vi "PDP.vi"() -> ()   [LabVIEW 2010]
doc: "This VI represents about 90% of the user interface, the remainder consisting of the various pop-up windows.\nA diagram of the NMR system is presented, with buttons to represent each component. Parameters may be changed by pressing one of these buttons, which results in messages being passed to one of several other, high-level VIs whose job it is to take action. After such action is taken, messages may be passed back to this VI, indicating new data to be displayed on the front panel."
uses:
  PDP Global.vi
  TPS Global.vi
  <vilib>/Utility/config.llb/Read Key (Path).vi
  TMC-Target_Motion_Control/TMC Global.vi
  <vilib>/Utility/config.llb/NI_LVConfig.lvlib
panel:
  in  "Case Constant\n(See Context Help)":bool
  out "Collector Temp":dbl=9.54 format="%.1f"
  in  "RF Off":bool
  in  "RF On":bool
  in  "Mon. Time":i32=30
  in  "He4 Range":i32(ring)=2 items=["X 1", "X 0.1", "X 0.01", "X 0.001"]
  out "Polysub Signal":cluster{"x-Axis":dbl[], "Signal":dbl[]}(graph)
  out "CarbGlass":dbl=9.54
  out "Bottom Chip":dbl=9.54
  out "Top Chip":dbl=9.54
  out "NMR Tune Light":bool
  in  "NMR Tune":bool
  out "Clear Message Time":i32
  in  "DC Convert":bool
  out "Vacuum Pressure":dbl format="%.2e"
  out "Bot Plat (K)":dbl=nan format="%.1f"
  out "Top Plat (K)":dbl=nan format="%.1f"
  out "Motion Mask":bool
  in  "Submit Comment":bool
  out "DC Level (V)":dbl=9.54 format="%.3f"
  out "QMeter Temp":dbl=9.54 format="%.1f"
  in  "User Comment (press submit when done)":string
  out "HP Freq(GHz)":dbl=500.0 format="%.5f"
  out "Heater 2":bool
  in  "FM Offset (V)":dbl format="%.1f"
  in  "FM Amplitude (V)":dbl=3.0 format="%.1f"
  out "Power (mW)":dbl=500.0 format="%.3f"
  out "Freq (GHz)":dbl=500.0 format="%.3f"
  in  "Stop NMR Sweep":bool
  in  "Enable TCL Buttons":bool
  in  "NewEventFile":bool
  in  "NewBaseFile":bool
  out "LN2":dbl(slide) scale=0.0..100.0
  out "Magnet":dbl(slide) scale=0.0..100.0
  out "Separator Flow":dbl=10.0 format="%.1f"
  out "Main Flow":dbl=9.83 format="%.1f"
  in  "Beep on Update":bool
  out "Raw & Base":cluster{"x-Axis":dbl[], "Signal":dbl[]}[](graph)
  in  "Move Target":bool
  out "Encoder":dbl format="%.3f"
  out "Target Pos":i32(listbox)
  in  "5 min":bool
  out "History Plot":cluster{dbl, dbl}[](graph)
  out "Event Number":i32=-15
  in  "Scan Freq":i32=100
  in  "ScanSteps":i32=500
  in  "RF Power":i32=280
  in  "RF Mod":i32=400
  in  "Sweeps":i32=100
  in  "RF Freq":dbl=213.0 format="%.3f"
  in  "Yale Gain":i32(listbox)
  in  "Decrease":bool
  in  "Increase":bool
  in  "Up":bool
  in  "Down":bool
  in  "+1 hour":bool
  in  "30 min":bool
  in  "15 min":bool
  out "Polarization (%)":string="-13.06%"
  out "Monitor Light":bool
  in  "Monitor":bool
  out "Take Data Light":bool
  out "Pause Light":bool=TRUE
  out "QMeter":string="Bot Proton NH3"
  in  "Error":bool
  out "3He Pressure":dbl=9.83 format="%.3f"
  out "4He Pressure":dbl=-0.06 format="%.3f"
  in  "Magnet Lockout":bool
  in  "Heater Delay Done":dbl=2993221584.8599997 format="%.2f"
  out "Heater Delay":i8
  in  "To Zero":bool
  in  "Hold":bool
  in  "To Setpoint":bool
  in  "Switch Heater Off":bool
  out "Timestamp":string="06May1999  19h28m14s"
  in  "Init QCA":bool
  out "PolyFit Area (arb units)":dbl=-14.751 format="%.8f"
  out "User Message":string="Message: 23Jul2001  15h39m59s\nQCA Module Started"
  in  "Cal. Const.":dbl=0.64413 format="%.6f"
  in  "5T Superconducting Magnet":T1={"Current (A)"=77.15, "Witness (mT)"=77.15, "Field (T)"=77.15} {"Field (T)" format="%.2f"; "Witness (mT)" format="%.3f"; "Current (A)" format="%.3f"}
  out "Update At (sec)":i32=2147483647
  out "Next Update":i32=1151566443
  in  "Baseline":bool
  out "Heater 1":bool
  out "Magnet Power Supply":T2={"Current (A):"=0.0, "Voltage (V):"=-0.01, "Setpoint (A):"=77.15, "Rate (A/min):"=0.3, "Heater Status"="Persistent Mode", "Status:"=enum."Hold"} {"Rate (A/min):" format="%.3f"; "Setpoint (A):" format="%.3f"; "Voltage (V):" format="%.3f"; "Current (A):" format="%.3f"}
  out "Subtracted Signal & PolyFit Curve":cluster{"x-Axis":dbl[], "Signal":dbl[]}[](graph)
  out "3He Temp":dbl=1.023 format="%.2f"
  out "4He Temp":dbl=nan format="%.2f"
  in  "Save Channel List":bool
  in  "Switch Heater On":bool
  in  "Rate (A/min)":dbl=0.5 format="%.2f"
  in  "SetPoint (A)":dbl=77.085 format="%.3f"
  in  "NMR Channel":i32(listbox)
  in  "Previous Messages":u16(ring)
  in  "Take Data":bool
  in  "One Point":bool
  in  "Pause":bool
  # "Data for Last Event Displayed:"
  # "RF Output"
  # "X-Axis"
  # "-->"
  # "Y-Axis"
  # "<--"
  # "Temp (K)"
  # "Press (Torr)"
  # "Range"
  # "4He"
  # "3He"
  # "Top"
  # "Bottom"
  # "Chip (W)"
  # "Plat (K)"
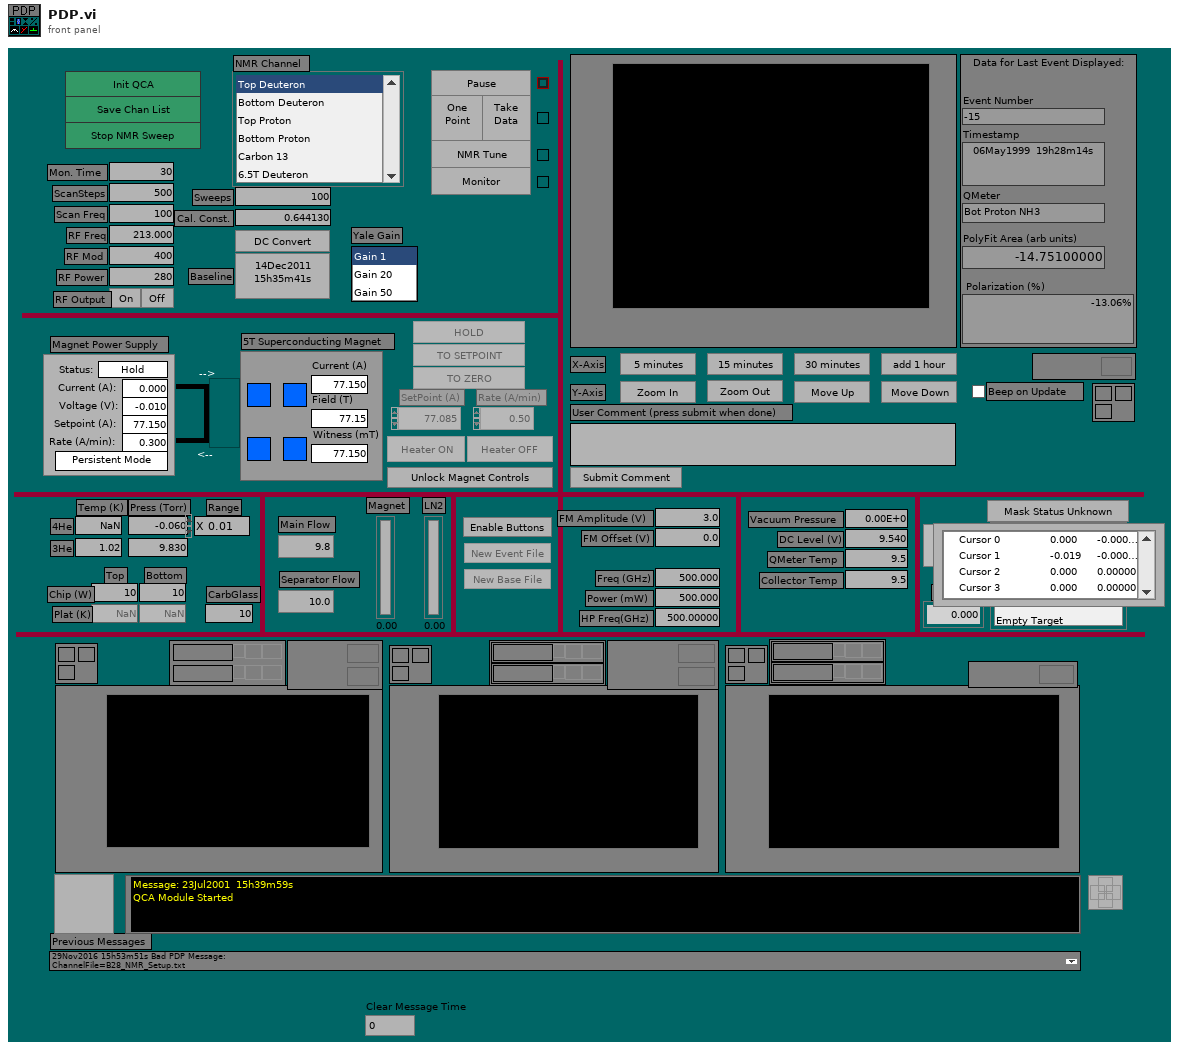
[diagram p1: front panel]
types:
  T1 = cluster{"Current (A)":dbl, "Witness (mT)":dbl, "Field (T)":dbl}
  T2 = cluster{"Current (A):":dbl, "Voltage (V):":dbl, "Setpoint (A):":dbl, "Rate (A/min):":dbl, "Heater Status":string, "Status:":enum16{"Hold", "To Setpoint", "To Zero", "Clamped"}}
  T3 = enum16{"No Message", "Bad Message", "RFFreq=", "RFMod=", "RFPower=", "QMeterName=", "YaleGain=", "ScanSweeps=", "ScanSteps=", "ScanFreq=", "Material=", "Baseline=", "CalConst=", "MonitorDelay=", "Channel=", "Channels=", "QCAPause", "QCATakeData", "QCANMRTune", "QCAMonitor", "Timer=", "LeadCurrent=", "LeadVoltage=", "MagCurrent=", "MagField=", "MagStatus=", "Setpoint=", "Setrate=", "HeaterDelay=", "Heater=", "HeaterDialog", "MagRemote", "MagLocal", "SendHe4Range", "uWaveFreq=", "uWavePower=", "BellowsPos=", "Event=", "Beep", "Message=", "Warning=", "Error=", "Address=", "Stop"}
  T4 = typedef "NI_LVConfig.lvlib/Config Data RefNum.ctl" = refnum<k1>
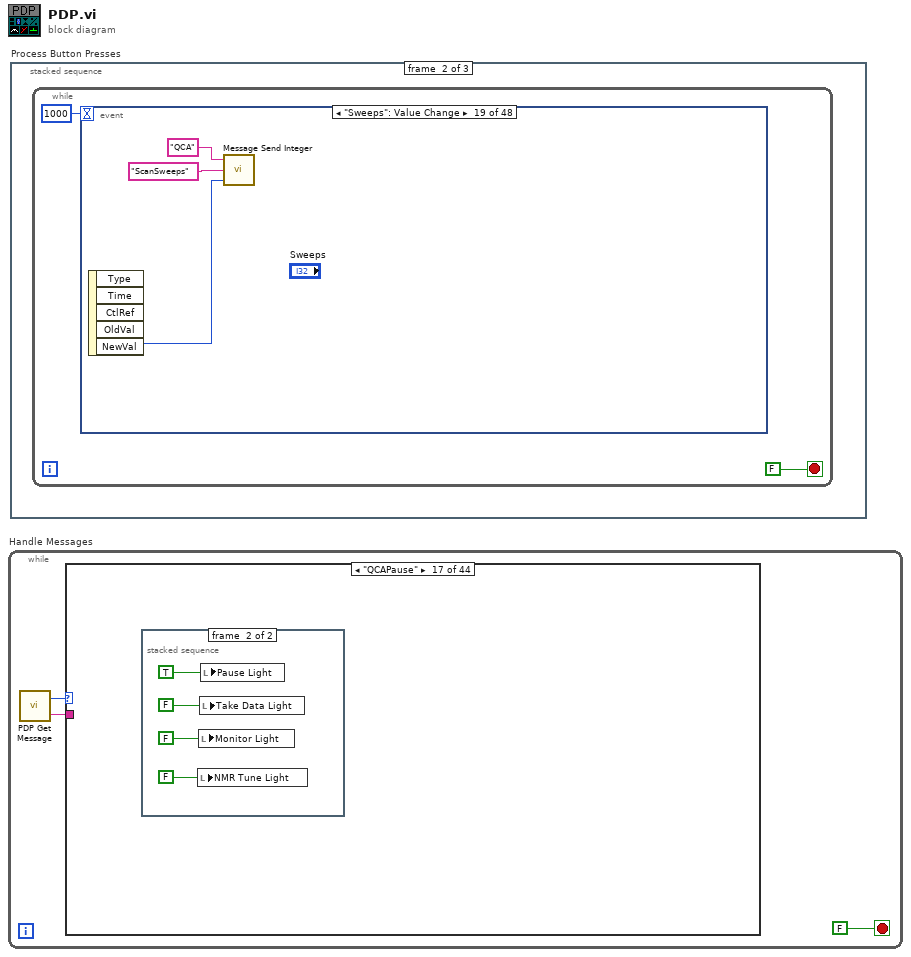
[diagram p0: block diagram]
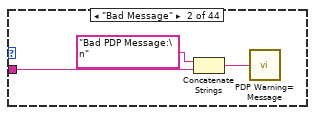
[diagram p3: hidden frame]
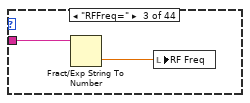
[diagram p4: hidden frame]
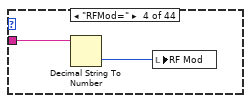
[diagram p5: hidden frame]
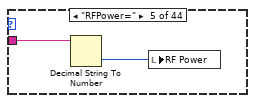
[diagram p6: hidden frame]
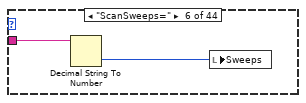
[diagram p7: hidden frame]
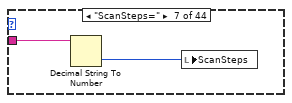
[diagram p8: hidden frame]
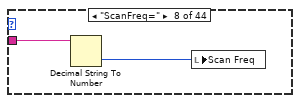
[diagram p9: hidden frame]
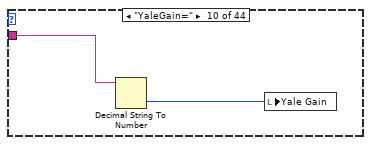
[diagram p11: hidden frame]
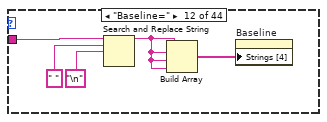
[diagram p13: hidden frame]
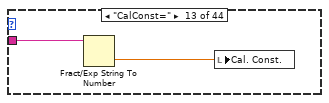
[diagram p14: hidden frame]
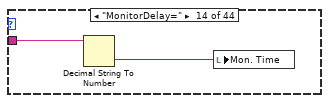
[diagram p15: hidden frame]
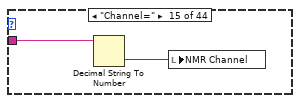
[diagram p16: hidden frame]
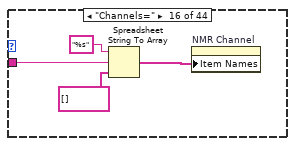
[diagram p17: hidden frame]
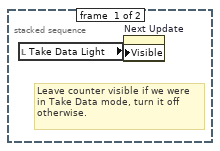
[diagram p18: hidden frame]
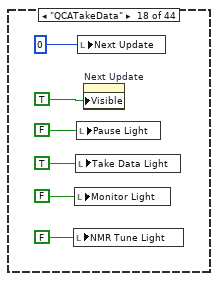
[diagram p19: hidden frame]
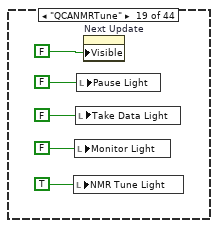
[diagram p20: hidden frame]
diagram:
  n1 = while "Handle Messages" {
    stop <- FALSE stop-if-true
    n2 = call "PDP Get Message.vi"() -> ("PDP Message Type"=w2:T3, "Text"=w3:string)  [unwired: 1 in]
    n3 = case shown="\"QCAPause\"" w2 {
      tunnel: w3 -> [_ w4 w8 w10 w12 w14 w16 w18 _ w20 _ w24 w27 w29 w31 w32 _ _ _ _ w61 w62 w66 w70 w74 w79 w83 w87 w94 w102 _ _ _ _ w126 w128 w130 w131 _ w396 w410 w425 w438 _]
      frame "No Message" {
      }
      frame "Bad Message" {
        n4 = Concatenate Strings("Bad PDP Message:\n" ("Message"), w4) -> (w5:string)
        n5 = call "PDP Warning= Message.vi"("Message"=w5) -> ()
      }
      frame "RFFreq=" {
        n6 = Fract/Exp String To Number(string=w8) -> (number=w7:dbl)  [unwired: 3 in, 1 out]
        n7 = local write "RF Freq"(w7) -> ()
      }
      frame "RFMod=" {
        n8 = Decimal String To Number(string=w10) -> (number=w9:i32)  [unwired: 2 in, 1 out]
        n9 = local write "RF Mod"(w9) -> ()
      }
      frame "RFPower=" {
        n10 = Decimal String To Number(string=w12) -> (number=w11:i32)  [unwired: 2 in, 1 out]
        n11 = local write "RF Power"(w11) -> ()
      }
      frame "ScanSweeps=" {
        n12 = Decimal String To Number(string=w14) -> (number=w13:i32)  [unwired: 2 in, 1 out]
        n13 = local write "Sweeps"(w13) -> ()
      }
      frame "ScanSteps=" {
        n14 = Decimal String To Number(string=w16) -> (number=w15:i32)  [unwired: 2 in, 1 out]
        n15 = local write "ScanSteps"(w15) -> ()
      }
      frame "ScanFreq=" {
        n16 = Decimal String To Number(string=w18) -> (number=w17:i32)  [unwired: 2 in, 1 out]
        n17 = local write "Scan Freq"(w17) -> ()
      }
      frame "QMeterName=" {
      }
      frame "YaleGain=" {
        n18 = Decimal String To Number(string=w20) -> (number=w19:i32)  [unwired: 2 in, 1 out]
        n19 = local write "Yale Gain"(w19) -> ()
      }
      frame "Material=" {
      }
      frame "Baseline=" {
        n20 = Search and Replace String(input string=w24, search string=" ", replace string="\n" ("replace string (\"\")")) -> (result string=w21:string)  [unwired: 5 in, 3 out]
        n21 = Build Array(w21, w21, w21, w21) -> (w25:string[])
        n22 = property on="Baseline" class="Bool"("Strings [4]"=w25) -> ()  [unwired: 2 in, 2 out]
      }
      frame "CalConst=" {
        n23 = Fract/Exp String To Number(string=w27) -> (number=w26:dbl)  [unwired: 3 in, 1 out]
        n24 = local write "Cal. Const."(w26) -> ()
      }
      frame "MonitorDelay=" {
        n25 = Decimal String To Number(string=w29) -> (number=w28:i32)  [unwired: 2 in, 1 out]
        n26 = local write "Mon. Time"(w28) -> ()
      }
      frame "Channel=" {
        n27 = Decimal String To Number(string=w31) -> (number=w30:i32)  [unwired: 2 in, 1 out]
        n28 = local write "NMR Channel"(w30) -> ()
      }
      frame "Channels=" {
        n29 = Spreadsheet String To Array(format string="%s", spreadsheet string=w32, array type (2D Dbl)=string[] []) -> (array=w34:string[])  [unwired: 1 in]
        n30 = property on="NMR Channel" class="LstBox (strict)"("Item Names"=w34) -> ()  [unwired: 2 in, 2 out]
      }
      frame "QCAPause" {
        n31 = stacked-sequence {
          frame #0 {
            # "Leave counter visible if we were\nin Take Data mode, turn it off\notherwise."
            n32 = local read "Take Data Light"() -> (w36:bool)
            n33 = property on="Next Update" class="DigNum (strict)"("Visible"=w36) -> ()  [unwired: 2 in, 2 out]
          }
          frame #1 {
            n34 = local write "NMR Tune Light"(FALSE ("NMR Tune Light")) -> ()
            n35 = local write "Monitor Light"(FALSE ("Cont Sweep Light")) -> ()
            n36 = local write "Take Data Light"(FALSE ("Take Data Light")) -> ()
            n37 = local write "Pause Light"(TRUE ("Pause Light")) -> ()
          }
        }
      }
      frame "QCATakeData" {
        n38 = local write "NMR Tune Light"(FALSE ("NMR Tune Light")) -> ()
        n39 = local write "Monitor Light"(FALSE ("Cont Sweep Light")) -> ()
        n40 = local write "Take Data Light"(TRUE ("Take Data Light")) -> ()
        n41 = local write "Pause Light"(FALSE ("Pause Light")) -> ()
        n42 = local write "Next Update"(0 ("Next Update")) -> ()
        n43 = property on="Next Update" class="DigNum (strict)"("Visible"=TRUE) -> ()  [unwired: 2 in, 2 out]
      }
      frame "QCANMRTune" {
        n44 = local write "NMR Tune Light"(TRUE ("NMR Tune Light")) -> ()
        n45 = local write "Monitor Light"(FALSE ("Cont Sweep Light")) -> ()
        n46 = local write "Take Data Light"(FALSE ("Take Data Light")) -> ()
        n47 = local write "Pause Light"(FALSE ("Pause Light")) -> ()
        n48 = property on="Next Update" class="DigNum (strict)"("Visible"=FALSE) -> ()  [unwired: 2 in, 2 out]
      }
      frame "QCAMonitor" {
        n49 = local write "NMR Tune Light"(FALSE ("NMR Tune Light")) -> ()
        n50 = local write "Monitor Light"(TRUE ("Cont Sweep Light")) -> ()
        n51 = local write "Take Data Light"(FALSE ("Take Data Light")) -> ()
        n52 = local write "Pause Light"(FALSE ("Pause Light")) -> ()
        n53 = local write "Next Update"(0 ("Next Update")) -> ()
        n54 = property on="Next Update" class="DigNum (strict)"("Visible"=TRUE) -> ()  [unwired: 2 in, 2 out]
      }
      frame "Timer=" {
        n55 = Decimal String To Number(string=w61) -> (number=w59:i32)  [unwired: 2 in, 1 out]
        n56 = call "Get UNIX Time.vi"() -> ("UNIX seconds"=w60:i32)
        n57 = Add(x=w59, y=w60) -> (x+y=→"Update At (sec)":i32)
      }
      frame "LeadCurrent=" {
        n58 = Fract/Exp String To Number(string=w62) -> (number=w65:dbl)  [unwired: 3 in, 1 out]
        n59 = local read "Magnet Power Supply"() -> (w63:T2)
        n60 = Bundle By Name(cluster=w63, "Current (A):"=w65) -> (w64:T2)
        n61 = local write "Magnet Power Supply"(w64) -> ()
      }
      frame "LeadVoltage=" {
        n62 = Fract/Exp String To Number(string=w66) -> (number=w69:dbl)  [unwired: 3 in, 1 out]
        n63 = local read "Magnet Power Supply"() -> (w67:T2)
        n64 = Bundle By Name(cluster=w67, "Voltage (V):"=w69) -> (w68:T2)
        n65 = local write "Magnet Power Supply"(w68) -> ()
      }
      frame "MagCurrent=" {
        n66 = Fract/Exp String To Number(string=w70) -> (number=w71:dbl)  [unwired: 3 in, 1 out]
        n67 = local read "5T Superconducting Magnet"() -> (w73:T1)
        n68 = Bundle By Name(cluster=w73, "Current (A)"=w71) -> (w72:T1)
        n69 = local write "5T Superconducting Magnet"(w72) -> ()
      }
      frame "MagField=" {
        n70 = Fract/Exp String To Number(string=w74) -> (number=w75:dbl)  [unwired: 3 in, 1 out]
        n71 = local read "5T Superconducting Magnet"() -> (w77:T1)
        n72 = Bundle By Name(cluster=w77, "Field (T)"=w75) -> (w76:T1)
        n73 = local write "5T Superconducting Magnet"(w76) -> ()
      }
      frame "MagStatus=" {
        n74 = Decimal String To Number(string=w79) -> (number=w78:i32)  [unwired: 2 in, 1 out]
        n75 = local read "Magnet Power Supply"() -> (w80:T2)
        n76 = Bundle By Name(cluster=w80, "Status:"=w78) -> (→"Magnet Power Supply":T2)
      }
      frame "Setpoint=" {
        n77 = Fract/Exp String To Number(string=w83) -> (number=w82:dbl)  [unwired: 3 in, 1 out]
        n78 = local write "SetPoint (A)"(w82) -> ()
        n79 = global write "PDP Global.vi" "Setpoint"(w82) -> ()
        n80 = local read "Magnet Power Supply"() -> (w84:T2)
        n81 = Bundle By Name(cluster=w84, "Setpoint (A):"=w82) -> (w85:T2)
        n82 = local write "Magnet Power Supply"(w85) -> ()
      }
      frame "Setrate=" {
        n83 = Fract/Exp String To Number(string=w87) -> (number=w86:dbl)  [unwired: 3 in, 1 out]
        n84 = local write "Rate (A/min)"(w86) -> ()
        n85 = global write "PDP Global.vi" "Setrate"(w86) -> ()
        n86 = local read "Magnet Power Supply"() -> (w88:T2)
        n87 = Bundle By Name(cluster=w88, "Rate (A/min):"=w86) -> (w89:T2)
        n88 = local write "Magnet Power Supply"(w89) -> ()
      }
      frame "HeaterDelay=" {
        n89 = Decimal String To Number(string=w94) -> (number=w91:i32)  [unwired: 2 in, 1 out]
        n90 = Get Date/Time In Seconds() -> (seconds since 1Jan1904=w90:timestamp)
        n91 = To Double Precision Float(number=w90) -> (double precision float=w93:dbl)
        n92 = Add(x=w91, y=w93) -> (x+y=w92:dbl)
        n93 = stacked-sequence {
          tunnel: w92 -> [w96 _]
          tunnel: w91 -> [w95 _]
          frame #0 {
            n94 = local write "Heater Delay Done"(w96) -> ()
            n95 = local write "Heater Delay"(w95) -> ()
          }
          frame #1 {
            n96 = property on="Switch Heater On" class="Bool"("Visible"=FALSE) -> ()  [unwired: 2 in, 2 out]
            n97 = property on="Switch Heater Off" class="Bool"("Visible"=FALSE) -> ()  [unwired: 2 in, 2 out]
            n98 = property on="Heater Delay" class="DigNum (strict)"("Visible"=TRUE) -> ()  [unwired: 2 in, 2 out]
          }
        }
      }
      frame "Heater=" {
        n99 = To Upper Case(1:w102) -> (0:w100:string)
        n100 = Equal?(x="ON", y=w100) -> (x = y?=w101:bool)
        "Heater 1" <- w101
        "Heater 2" <- w101
        n101 = Select(t="Driven Mode", s=w101, f="Persistent Mode") -> (s? t:f=w108:string)
        n102 = local read "Magnet Power Supply"() -> (w103:T2)
        n103 = Bundle By Name(cluster=w103, "Heater Status"=w108) -> (w104:T2)
        n104 = local write "Magnet Power Supply"(w104) -> ()
      }
      frame "HeaterDialog" {
        n105 = Two Button Dialog(message="Are you sure you want to turn the switch heater on? ", 1:"Cancel - No Change" ("F button name (\"Cancel\")"), 2:"Turn Heater On" ("T button name (\"OK\")")) -> (T button?=w109:bool)
        n106 = case shown="True" w109 {
          frame False {
          }
          frame True {
            n107 = call "Message Send Text.vi"("Value"="On,Confirm" ("Message"), "Parameter"="Heater", "Destination"="SMC") -> ()
          }
        }
      }
      frame "MagRemote" {
        w116 = u8 0
        n108 = Build Array("Lock Magnet Controls") -> (w118:string[])
        n109 = property on="SetPoint (A)" class="DigNum (strict)"("Disabled"=w116) -> ()  [unwired: 2 in, 2 out]
        n110 = property on="Switch Heater On" class="Bool"("Disabled"=w116) -> ()  [unwired: 2 in, 2 out]
        n111 = property on="Switch Heater Off" class="Bool"("Disabled"=w116) -> ()  [unwired: 2 in, 2 out]
        n112 = property on="Magnet Lockout" class="Bool"("Strings [4]"=w118) -> ()  [unwired: 2 in, 2 out]
        n113 = property on="Rate (A/min)" class="DigNum (strict)"("Disabled"=w116) -> ()  [unwired: 2 in, 2 out]
        n114 = property on="Hold" class="Bool"("Disabled"=w116) -> ()  [unwired: 2 in, 2 out]
        n115 = property on="To Setpoint" class="Bool"("Disabled"=w116) -> ()  [unwired: 2 in, 2 out]
        n116 = property on="To Zero" class="Bool"("Disabled"=w116) -> ()  [unwired: 2 in, 2 out]
      }
      frame "MagLocal" {
        w119 = u8 2
        n117 = Build Array("Unlock Magnet Controls") -> (w121:string[])
        n118 = property on="SetPoint (A)" class="DigNum (strict)"("Disabled"=w119) -> ()  [unwired: 2 in, 2 out]
        n119 = property on="Switch Heater On" class="Bool"("Disabled"=w119) -> ()  [unwired: 2 in, 2 out]
        n120 = property on="Switch Heater Off" class="Bool"("Disabled"=w119) -> ()  [unwired: 2 in, 2 out]
        n121 = property on="Magnet Lockout" class="Bool"("Strings [4]"=w121) -> ()  [unwired: 2 in, 2 out]
        n122 = property on="Rate (A/min)" class="DigNum (strict)"("Disabled"=w119) -> ()  [unwired: 2 in, 2 out]
        n123 = property on="Hold" class="Bool"("Disabled"=w119) -> ()  [unwired: 2 in, 2 out]
        n124 = property on="To Setpoint" class="Bool"("Disabled"=w119) -> ()  [unwired: 2 in, 2 out]
        n125 = property on="To Zero" class="Bool"("Disabled"=w119) -> ()  [unwired: 2 in, 2 out]
      }
      frame "SendHe4Range" {
        n126 = call "Message Send Integer.vi"("Value"="He4 Range", "Parameter"="He4Range", "Destination"="TTM") -> ()
      }
      frame "uWaveFreq=" {
        n127 = Fract/Exp String To Number(string=w126) -> (number=w125:dbl)  [unwired: 3 in, 1 out]
        n128 = local write "Freq (GHz)"(w125) -> ()
      }
      frame "uWavePower=" {
        n129 = Fract/Exp String To Number(string=w128) -> (number=w127:dbl)  [unwired: 3 in, 1 out]
        n130 = local write "Power (mW)"(w127) -> ()
      }
      frame "BellowsPos=" {
        n131 = Fract/Exp String To Number(string=w130) -> (number=w129:dbl)  [unwired: 3 in, 1 out]
        n132 = local write "HP Freq(GHz)"(w129) -> ()
      }
      frame "Event=" {
        n133 = Unflatten From String(type=string[][] [], binary string=w131) -> (value=w133:string[][])  [unwired: 3 in, 2 out]
        n134 = stacked-sequence {
          tunnel: w133 -> [w144 w172 w193 w200 w203 w207 w234 w237 w242 w246 w250 w255 w266 w275 w278 w282 w286 w290 w296 w302 w306 w310 w316 w322 w326 w335 w344 w348 w352 w359 w374 _ w391]
          frame #0 {
            # "Set the X axis of the signal plots."
            n135 = call "Text Get Event Fragment.vi"("Event"=w144, "Fragment Type"="RFFreq") -> ("Fragment"=w149:string)  [unwired: 1 out]
            n136 = call "Text Get Event Fragment.vi"("Event"=w144, "Fragment Type"="RFMod") -> ("Fragment"=w150:string)  [unwired: 1 out]
            n137 = call "Text Get Event Fragment.vi"("Event"=w144, "Fragment Type"="ScanSteps") -> ("Fragment"=w146:string)  [unwired: 1 out]
            n138 = global read "PDP Global.vi" "Last Mod"() -> (w140:dbl)
            n139 = global read "PDP Global.vi" "Last Freq"() -> (w143:dbl)
            n140 = global read "PDP Global.vi" "Last Steps"() -> (w141:i32)
            n141 = Fract/Exp String To Number(string=w149) -> (number=w142:dbl)  [unwired: 3 in, 1 out]
            n142 = Decimal String To Number(string=w150) -> (number=w148:i32)  [unwired: 2 in, 1 out]
            n143 = Decimal String To Number(string=w146) -> (number=w138:i32)  [unwired: 2 in, 1 out]
            n144 = Divide(x=w148, y=1000) -> (x/y=w139:dbl)
            n145 = Not Equal?(x=w143, y=w142) -> (x != y?=w135:bool)
            n146 = Not Equal?(x=w140, y=w139) -> (x != y?=w136:bool)
            n147 = Not Equal?(x=w141, y=w138) -> (x != y?=w137:bool)
            n148 = Compound Arithmetic op=OR(w135, w136, w137) -> (w134:bool)
            n149 = case shown="True" w134 {
              tunnel: w138 -> [_ w155]
              tunnel: w139 -> [_ w154]
              tunnel: w142 -> [_ w153]
              frame False {
              }
              frame True {
                n150 = global write "PDP Global.vi" "Last Mod"(w154) -> ()
                n151 = global write "PDP Global.vi" "Last Freq"(w153) -> ()
                n152 = global write "PDP Global.vi" "Last Steps"(w155) -> ()
                n153 = for {
                  N: w155 -> [_]
                  tunnel: [w163] -> w158 mode=indexing
                  i -> [w163]
                }
                n154 = Multiply(x=w158, y=2) -> (x*y=w159:i32[])
                n155 = Divide(x=w159, y=w155) -> (x/y=w162:dbl[])
                n156 = Decrement(x=w162) -> (x-1=w156:dbl[])
                n157 = Multiply(x=w154, y=w156) -> (x*y=w161:dbl[])
                n158 = Add(x=w153, y=w161) -> (x+y=w160:dbl[])
                n159 = global write "PDP Global.vi" "x-Axis"(w160) -> ()
              }
            }
          }
          frame #1 {
            # "Display the Raw Signal and the Baseline Signal."
            n160 = call "Text Get Event Fragment.vi"("Event"=w172, "Fragment Type"="RawSignal") -> ("Fragment"=w171:string)  [unwired: 1 out]
            n161 = call "Text Get Event Fragment.vi"("Event"=w172, "Fragment Type"="BaseSignal") -> ("Fragment"=w170:string)  [unwired: 1 out]
            n162 = global read "PDP Global.vi" "x-Axis"() -> (w168:dbl[])
            n163 = call "String 2 Signal.vi"("String"=w171) -> ("Signal"=w165:dbl[])
            n164 = call "String 2 Signal.vi"("String"=w170) -> ("Signal"=w167:dbl[])
            n165 = Array Size(array=w167) -> (size(s)=w169:i32)
            n166 = Greater Than 0?(x=w169) -> (x > 0?=w164:bool)
            n167 = case shown="True" w164 {
              tunnel: w168 -> [w178 w179]
              tunnel: w167 -> [_ w184]
              tunnel: [w175 w181] -> w166
              tunnel: w165 -> [w177 w180]
              frame False {
                n168 = Bundle("x-Axis"=w178, "Signal"=w177) -> (w176:cluster{"x-Axis":dbl[], "Signal":dbl[]})  [unwired: 1 in]
                n169 = Build Array(w176) -> (w175:cluster{"x-Axis":dbl[], "Signal":dbl[]}[])
              }
              frame True {
                n170 = Bundle("x-Axis"=w179, "Signal"=w180) -> (w183:cluster{"x-Axis":dbl[], "Signal":dbl[]})  [unwired: 1 in]
                n171 = Bundle("x-Axis"=w179, "Signal"=w184) -> (w182:cluster{"x-Axis":dbl[], "Signal":dbl[]})  [unwired: 1 in]
                n172 = Build Array(w183, w182) -> (w181:cluster{"x-Axis":dbl[], "Signal":dbl[]}[])
              }
            }
            "Raw & Base" <- w166
          }
          frame #2 {
            # "Display the Subtracted Signal and the Polyfit Curve."
            n173 = call "Text Get Event Fragment.vi"("Event"=w193, "Fragment Type"="SubSignal") -> ("Fragment"=w191:string)  [unwired: 1 out]
            n174 = call "Text Get Event Fragment.vi"("Event"=w193, "Fragment Type"="PolyCurve") -> ("Fragment"=w192:string)  [unwired: 1 out]
            n175 = global read "PDP Global.vi" "x-Axis"() -> (w188:dbl[])
            n176 = call "String 2 Signal.vi"("String"=w191) -> ("Signal"=w185:dbl[])
            n177 = call "String 2 Signal.vi"("String"=w192) -> ("Signal"=w189:dbl[])
            n178 = Bundle("x-Axis"=w188, "Signal"=w185) -> (w186:cluster{"x-Axis":dbl[], "Signal":dbl[]})  [unwired: 1 in]
            n179 = Bundle("x-Axis"=w188, "Signal"=w189) -> (w187:cluster{"x-Axis":dbl[], "Signal":dbl[]})  [unwired: 1 in]
            n180 = Build Array(w186, w187) -> (→"Subtracted Signal & PolyFit Curve":cluster{"x-Axis":dbl[], "Signal":dbl[]}[])
          }
          frame #3 {
            # "Display the Polysubtracted Signal."
            n181 = call "Text Get Event Fragment.vi"("Event"=w200, "Fragment Type"="PolySignal") -> ("Fragment"=w196:string)  [unwired: 1 out]
            n182 = global read "PDP Global.vi" "x-Axis"() -> (w199:dbl[])
            n183 = call "String 2 Signal.vi"("String"=w196) -> ("Signal"=w197:dbl[])
            n184 = Bundle("x-Axis"=w199, "Signal"=w197) -> (→"Polysub Signal":cluster{"x-Axis":dbl[], "Signal":dbl[]})  [unwired: 1 in]
          }
          frame #4 {
            # "Display the Polysubtracted Signal."
            n185 = call "Text Get Event Fragment.vi"("Event"=w203, "Fragment Type"="Area") -> ("Fragment"=w204:string)  [unwired: 1 out]
            n186 = Fract/Exp String To Number(string=w204) -> (number=→"PolyFit Area (arb units)":dbl)  [unwired: 3 in, 1 out]
          }
          frame #5 {
            # "Display the Polysubtracted Signal."
            n187 = call "Text Get Event Fragment.vi"("Event"=w207, "Fragment Type"="Polarization") -> ("Fragment"=w213:string, "Found"=w206:bool)
            n188 = call "Text Get Event Fragment.vi"("Event"=w207, "Fragment Type"="EventNum") -> ("Fragment"=w209:string)  [unwired: 1 out]
            n189 = Decimal String To Number(string=w209) -> (number=w208:i32)  [unwired: 2 in, 1 out]
            n190 = Fract/Exp String To Number(string=w213) -> (number=w211:dbl)  [unwired: 3 in, 1 out]
            n191 = case shown="True" w206 {
              tunnel: w211 -> [_ w218]
              tunnel: w208 -> [_ w219]
              frame False {
                n192 = local write "Polarization (%)"("") -> ()
              }
              frame True {
                n193 = call "UNIX to LabVIEW.vi"("UNIX Time"=w219) -> ("LabVIEW Time"=w220:dbl)
                n194 = Absolute Value(x=w218) -> (abs(x)=w217:dbl)
                n195 = property on="History Plot" class="XYGraph (strict)"() -> ("X Scale.Range:Maximum"=w223:dbl, "X Scale.Range:Minimum"=w226:dbl)  [unwired: 2 in, 2 out]
                n196 = Less?(x=w217, y=101.0) -> (x < y?=w215:bool)
                n197 = Format Into String(format string="%+6.1f%", w218) -> (resulting string=→"Polarization (%)":string)  [unwired: 2 in, 1 out]
                n198 = case shown="True" w215 {
                  tunnel: w220 -> [_ w229]
                  tunnel: w218 -> [_ w228]
                  frame False {
                    # "Glitch Signal - don't plot in strip chart"
                  }
                  frame True {
                    n199 = local read "History Plot"() -> (w232:cluster{dbl, dbl}[])
                    n200 = Bundle("LabVIEW Time"=w229, w228) -> (w230:cluster{"LabVIEW Time":dbl, dbl})  [unwired: 1 in]
                    n201 = Build Array (concatenate)(w230, w232) -> (→"History Plot":cluster{"LabVIEW Time":dbl, dbl}[])
                  }
                }
                n202 = Subtract(x=w220, y=w223) -> (x-y=w227:dbl)
                n203 = Compound Arithmetic op=ADD(w227, w223) -> (w225:dbl)
                n204 = Compound Arithmetic op=ADD(w227, w226) -> (w224:dbl)
                n205 = property on="History Plot" class="XYGraph (strict)"("X Scale.Range:Maximum"=w225, "X Scale.Range:Minimum"=w224) -> ()  [unwired: 2 in, 2 out]
              }
            }
          }
          frame #6 {
            # "Display the Polysubtracted Signal."
            n206 = call "Text Get Event Fragment.vi"("Event"=w234, "Fragment Type"="QMeterName") -> ("Fragment"=→"QMeter":string)  [unwired: 1 out]
          }
          frame #7 {
            n207 = call "Text Get Event Fragment.vi"("Event"=w237, "Fragment Type"="EventNum") -> ("Fragment"=w238:string)  [unwired: 1 out]
            n208 = Decimal String To Number(string=w238) -> (number=w236:i32)  [unwired: 2 in, 1 out]
            "Event Number" <- w236
            n209 = call "UNIX to Timestamp.vi"("Seconds"=w236) -> ("Timestamp String"=→"Timestamp":string)
          }
          frame #8 {
            # "Display the Polysubtracted Signal."
            n210 = call "Text Get Event Fragment.vi"("Event"=w242, "Fragment Type"="He3Press") -> ("Fragment"=w243:string)  [unwired: 1 out]
            n211 = Fract/Exp String To Number(string=w243) -> (number=→"3He Pressure":dbl)  [unwired: 3 in, 1 out]
          }
          frame #9 {
            # "Display the Polysubtracted Signal."
            n212 = call "Text Get Event Fragment.vi"("Event"=w246, "Fragment Type"="He3Temp") -> ("Fragment"=w247:string)  [unwired: 1 out]
            n213 = Fract/Exp String To Number(string=w247) -> (number=→"3He Temp":dbl)  [unwired: 3 in, 1 out]
          }
          frame #10 {
            # "Display the Polysubtracted Signal."
            n214 = call "Text Get Event Fragment.vi"("Event"=w250, "Fragment Type"="He4Press") -> ("Fragment"=w251:string)  [unwired: 1 out]
            n215 = Fract/Exp String To Number(string=w251) -> (number=→"4He Pressure":dbl)  [unwired: 3 in, 1 out]
          }
          frame #11 {
            # "Display the Polysubtracted Signal."
            n216 = call "Text Get Event Fragment.vi"("Event"=w255, "Fragment Type"="He4Temp") -> ("Fragment"=w256:string, "Found"=w253:bool)
            n217 = Fract/Exp String To Number(string=w256) -> (number=w254:dbl)  [unwired: 3 in, 1 out]
            n218 = case shown="True" w253 {
              tunnel: w254 -> [_ w258]
              frame False {
              }
              frame True {
                "4He Temp" <- w258
              }
            }
          }
          frame #12 {
            # "Display the Polysubtracted Signal."
            n219 = call "Text Get Event Fragment.vi"("Event"=w266, "Fragment Type"="TopPlat") -> ("Fragment"=w261:string)  [unwired: 1 out]
            n220 = Fract/Exp String To Number(string=w261) -> (number=w260:dbl)  [unwired: 3 in, 1 out]
            "Top Plat (K)" <- w260
            n221 = Less?(x=w260, y=49.0) -> (x < y?=w265:bool)
            n222 = Select(t=2, s=w265, f=0) -> (s? t:f=w262:i32)
            n223 = property on="Top Plat (K)" class="DigNum (strict)"("Disabled"=w262) -> ()  [unwired: 2 in, 2 out]
          }
          frame #13 {
            # "Display the Polysubtracted Signal."
            n224 = call "Text Get Event Fragment.vi"("Event"=w275, "Fragment Type"="BotPlat") -> ("Fragment"=w271:string)  [unwired: 1 out]
            n225 = Fract/Exp String To Number(string=w271) -> (number=w268:dbl)  [unwired: 3 in, 1 out]
            "Bot Plat (K)" <- w268
            n226 = Less?(x=w268, y=49.0) -> (x < y?=w274:bool)
            n227 = Select(t=2, s=w274, f=0) -> (s? t:f=w269:i32)
            n228 = property on="Bot Plat (K)" class="DigNum (strict)"("Disabled"=w269) -> ()  [unwired: 2 in, 2 out]
          }
          frame #14 {
            # "Display the Polysubtracted Signal."
            n229 = call "Text Get Event Fragment.vi"("Event"=w278, "Fragment Type"="uWaveFreq") -> ("Fragment"=w279:string)  [unwired: 1 out]
            n230 = Fract/Exp String To Number(string=w279) -> (number=→"Freq (GHz)":dbl)  [unwired: 3 in, 1 out]
          }
          frame #15 {
            # "Display the Polysubtracted Signal."
            n231 = call "Text Get Event Fragment.vi"("Event"=w282, "Fragment Type"="uWavePower") -> ("Fragment"=w283:string)  [unwired: 1 out]
            n232 = Fract/Exp String To Number(string=w283) -> (number=→"Power (mW)":dbl)  [unwired: 3 in, 1 out]
          }
          frame #16 {
            # "Display the Polysubtracted Signal."
            n233 = call "Text Get Event Fragment.vi"("Event"=w286, "Fragment Type"="HPFreq") -> ("Fragment"=w287:string)  [unwired: 1 out]
            n234 = Fract/Exp String To Number(string=w287) -> (number=→"HP Freq(GHz)":dbl)  [unwired: 3 in, 1 out]
          }
          frame #17 {
            n235 = call "Text Get Event Fragment.vi"("Event"=w290, "Fragment Type"="MainFlow") -> ("Fragment"=w291:string)  [unwired: 1 out]
            n236 = Fract/Exp String To Number(string=w291) -> (number=→"Main Flow":dbl)  [unwired: 3 in, 1 out]
          }
          frame #18 {
            n237 = call "Text Get Event Fragment.vi"("Event"=w296, "Fragment Type"="SepFlow") -> ("Fragment"=w297:string)  [unwired: 1 out]
            n238 = Fract/Exp String To Number(string=w297) -> (number=w294:dbl)  [unwired: 3 in, 1 out]
            "Separator Flow" <- w294
            n239 = Less?(x=w294, y=7.0) -> (x < y?=w295:bool)
            n240 = property on="Separator Flow" class="DigNum (strict)"("Blinking"=w295) -> ()  [unwired: 2 in, 2 out]
          }
          frame #19 {
            n241 = call "Text Get Event Fragment.vi"("Event"=w302, "Fragment Type"="Collector") -> ("Fragment"=w303:string)  [unwired: 1 out]
            n242 = Fract/Exp String To Number(string=w303) -> (number=w300:dbl)  [unwired: 3 in, 1 out]
            "Collector Temp" <- w300
            n243 = Greater?(x=w300, y=35.0) -> (0:w299:bool)
            n244 = property on="Collector Temp" class="DigNum (strict)"("Blinking"=w299) -> ()  [unwired: 2 in, 2 out]
          }
          frame #20 {
            n245 = call "Text Get Event Fragment.vi"("Event"=w306, "Fragment Type"="MagLevel") -> ("Fragment"=w308:string)  [unwired: 1 out]
            n246 = Fract/Exp String To Number(string=w308) -> (number=→"Magnet":dbl)  [unwired: 3 in, 1 out]
          }
          frame #21 {
            n247 = call "Text Get Event Fragment.vi"("Event"=w310, "Fragment Type"="LN2Level") -> ("Fragment"=w311:string)  [unwired: 1 out]
            n248 = Fract/Exp String To Number(string=w311) -> (number=→"LN2":dbl)  [unwired: 3 in, 1 out]
          }
          frame #22 {
            n249 = call "Text Get Event Fragment.vi"("Event"=w316, "Fragment Type"="WitnessField") -> ("Fragment"=w317:string)  [unwired: 1 out]
            n250 = Fract/Exp String To Number(string=w317) -> (number=w314:dbl)  [unwired: 3 in, 1 out]
            n251 = Bundle By Name(cluster="5T Superconducting Magnet", "Witness (mT)"=w314) -> (w313:T1)
            n252 = local write "5T Superconducting Magnet"(w313) -> ()
          }
          frame #23 {
            n253 = call "Text Get Event Fragment.vi"("Event"=w322, "Fragment Type"="MagField") -> ("Fragment"=w323:string)  [unwired: 1 out]
            n254 = local read "5T Superconducting Magnet"() -> (w319:T1)
            n255 = Fract/Exp String To Number(string=w323) -> (number=w321:dbl)  [unwired: 3 in, 1 out]
            n256 = Bundle By Name(cluster=w319, "Field (T)"=w321) -> (w320:T1)
            n257 = local write "5T Superconducting Magnet"(w320) -> ()
          }
          frame #24 {
            n258 = call "Text Get Event Fragment.vi"("Event"=w326, "Fragment Type"="QMeterTemp") -> ("Fragment"=w327:string)  [unwired: 1 out]
            n259 = Fract/Exp String To Number(string=w327) -> (number=→"QMeter Temp":dbl)  [unwired: 3 in, 1 out]
          }
          frame #25 {
            w334 = 1300  # Liquid Threshold
            n260 = call "Text Get Event Fragment.vi"("Event"=w335, "Fragment Type"="TopChip") -> ("Fragment"=w336:string)  [unwired: 1 out]
            n261 = Fract/Exp String To Number(string=w336) -> (number=w333:dbl)  [unwired: 3 in, 1 out]
            "Top Chip" <- w333
            n262 = Greater?(x=w333, y=w334) -> (0:w330:bool)
            n263 = Select(t=u32 4372735, s=w330, f=u32 11776947) -> (s? t:f=w329:u32)
            n264 = property on="Top Chip" class="DigNum (strict)"("Numeric Text.Text Colors:BG Color"=w329) -> ()  [unwired: 2 in, 2 out]
          }
          frame #26 {
            w343 = 1300  # Liquid Threshold
            n265 = call "Text Get Event Fragment.vi"("Event"=w344, "Fragment Type"="BottomChip") -> ("Fragment"=w345:string)  [unwired: 1 out]
            n266 = Fract/Exp String To Number(string=w345) -> (number=w342:dbl)  [unwired: 3 in, 1 out]
            "Bottom Chip" <- w342
            n267 = Greater?(x=w342, y=w343) -> (0:w339:bool)
            n268 = Select(t=u32 4372735, s=w339, f=u32 11776947) -> (s? t:f=w338:u32)
            n269 = property on="Bottom Chip" class="DigNum (strict)"("Numeric Text.Text Colors:BG Color"=w338) -> ()  [unwired: 2 in, 2 out]
          }
          frame #27 {
            n270 = call "Text Get Event Fragment.vi"("Event"=w348, "Fragment Type"="CarbonGlass") -> ("Fragment"=w349:string)  [unwired: 1 out]
            n271 = Fract/Exp String To Number(string=w349) -> (number=→"CarbGlass":dbl)  [unwired: 3 in, 1 out]
          }
          frame #28 {
            n272 = call "Text Get Event Fragment.vi"("Event"=w352, "Fragment Type"="DCLevel") -> ("Fragment"=w353:string)  [unwired: 1 out]
            n273 = Fract/Exp String To Number(string=w353) -> (number=→"DC Level (V)":dbl)  [unwired: 3 in, 1 out]
          }
          frame #29 {
            n274 = call "Text Get Event Fragment.vi"("Event"=w359, "Fragment Type"="VacPress") -> ("Fragment"=w360:string)  [unwired: 1 out]
            n275 = Fract/Exp String To Number(string=w360) -> (number=w358:dbl)  [unwired: 3 in, 1 out]
            n276 = Power Of 10(x=w358) -> (10^x=w357:dbl)
            "Vacuum Pressure" <- w357
            n277 = Greater?(x=w357, y=5e-05) -> (0:w355:bool)
            n278 = property on="Vacuum Pressure" class="DigNum (strict)"("Blinking"=w355) -> ()  [unwired: 2 in, 2 out]
          }
          frame #30 {
            n279 = call "Text Get Event Fragment.vi"("Event"=w374, "Fragment Type"="ISD3H002N") -> ("Fragment"=w375:string, "Found"=w362:bool)
            n280 = Decimal String To Number(string=w375) -> (number=w373:i32)  [unwired: 2 in, 1 out]
            n281 = Number To Boolean Array(number=w373) -> (Boolean array=w372:bool[])
            n282 = Number To Boolean Array(number=128) -> (Boolean array=w371:bool[])
            n283 = And(x=w372, y=w371) -> (x .and. y?=w369:bool[])
            n284 = Or Array Elements(Boolean array=w369) -> (logical OR=w368:bool)
            n285 = case shown="False" w362 {
              tunnel: w368 -> [w379 _]
              tunnel: [w378 "Mask Status Unknown"] -> w367
              tunnel: [w377 u32 11776947] -> w365
              frame True {
                n286 = case shown="False" w379 {
                  tunnel: [u32 65280 u32 16722506] -> w377
                  tunnel: ["OK to Move Target" "Do NOT Move Target!"] -> w378
                  frame True {
                  }
                  frame False {
                  }
                }
              }
              frame False {
              }
            }
            n287 = Bundle(w365, w365) -> (w364:cluster{u32, u32})  [unwired: 1 in]
            n288 = Build Array(w367) -> (w366:string[])
            n289 = Build Array(w364) -> (w363:cluster{u32, u32}[])
            n290 = property on="Motion Mask" class="Bool (strict)"("Strings [4]"=w366) -> ()  [unwired: 2 in, 2 out]
            n291 = property on="Motion Mask" class="Bool (strict)"("Colors [4]"=w363) -> ()  [unwired: 2 in, 2 out]
          }
          frame #31 {
            n292 = case shown="True" "Beep on Update" {
              frame False {
              }
              frame True {
                n293 = call <vilib>:"Beep.vi"() -> ()  [unwired: 12 in]
              }
            }
          }
          frame #32 {
            # "Tell the event builder that we're done."
            n294 = call "Text Get Event Fragment.vi"("Event"=w391, "Fragment Type"="EventNum") -> ("Fragment"=w389:string)  [unwired: 1 out]
            n295 = Decimal String To Number(string=w389) -> (number=w388:i32)  [unwired: 2 in, 1 out]
            n296 = call "TEB Processed= Message.vi"("Module Name"="PDP", "Event Number"=w388) -> ()
          }
        }
      }
      frame "Beep" {
        n297 = call <vilib>:"Beep.vi"() -> ()  [unwired: 12 in]
      }
      frame "Message=" {
        n298 = call "Get UNIX Time.vi"() -> ("UNIX seconds"=w393:i32)
        n299 = call "UNIX to Timestamp.vi"("Seconds"=w393) -> ("Timestamp String"=w405:string)
        n300 = Add(x=60, y=w393) -> (x+y=→"Clear Message Time":i32)
        n301 = property on="Previous Messages" class="Ring (strict)"() -> ("Strings []"=w399:string[])  [unwired: 2 in, 2 out]
        n302 = Format Into String(format string="Message: %s\n%s", w405, w396) -> (resulting string=w395:string)  [unwired: 2 in, 1 out]
        n303 = Format Into String(format string="%s %s", w405, w396) -> (resulting string=w404:string)  [unwired: 2 in, 1 out]
        n304 = Array Subset(array=w399, length=99) -> (w401:string[])  [unwired: 1 in]
        n305 = Build Array (concatenate)(w404, w401) -> (w402:string[])
        n306 = local write "User Message"(w395) -> ()
        n307 = call "PDP Log Message.vi"("Message"=w395) -> ()
        n308 = property on="Previous Messages" class="Ring (strict)"("Strings []"=w402) -> ()  [unwired: 2 in, 2 out]
        n309 = property on="User Message" class="Str"("Text.Text Colors:Text Color"=u32 65280) -> ()  [unwired: 2 in, 2 out]
      }
      frame "Warning=" {
        n310 = call "Get UNIX Time.vi"() -> ("UNIX seconds"=w407:i32)
        n311 = Add(x=180, y=w407) -> (x+y=w408:i32)
        n312 = call "UNIX to Timestamp.vi"("Seconds"=w407) -> ("Timestamp String"=w419:string)
        n313 = local write "Clear Message Time"(w408) -> ()
        n314 = property on="Previous Messages" class="Ring (strict)"() -> ("Strings []"=w413:string[])  [unwired: 2 in, 2 out]
        n315 = Format Into String(format string="Warning: %s\n%s", w419, w410) -> (resulting string=w409:string)  [unwired: 2 in, 1 out]
        n316 = Format Into String(format string="%s %s", w419, w410) -> (resulting string=w418:string)  [unwired: 2 in, 1 out]
        n317 = Array Subset(array=w413, length=99) -> (w415:string[])  [unwired: 1 in]
        n318 = Build Array (concatenate)(w418, w415) -> (w416:string[])
        n319 = local write "User Message"(w409) -> ()
        n320 = call "PDP Log Message.vi"("Message"=w409) -> ()
        n321 = property on="Previous Messages" class="Ring (strict)"("Strings []"=w416) -> ()  [unwired: 2 in, 2 out]
        n322 = call <vilib>:"Beep.vi"() -> ()  [unwired: 12 in]
        n323 = property on="User Message" class="Str"("Text.Text Colors:Text Color"=u32 16776960) -> ()  [unwired: 2 in, 2 out]
      }
      frame "Error=" {
        n324 = call "Get UNIX Time.vi"() -> ("UNIX seconds"=w421:i32)
        n325 = Add(x=300, y=w421) -> (x+y=w422:i32)
        n326 = call "UNIX to Timestamp.vi"("Seconds"=w421) -> ("Timestamp String"=w434:string)
        n327 = property on="Previous Messages" class="Ring (strict)"() -> ("Strings []"=w428:string[])  [unwired: 2 in, 2 out]
        n328 = local write "Clear Message Time"(w422) -> ()
        n329 = Format Into String(format string="Error: %s\n%s", w434, w425) -> (resulting string=w423:string)  [unwired: 2 in, 1 out]
        n330 = Format Into String(format string="%s %s", w434, w425) -> (resulting string=w433:string)  [unwired: 2 in, 1 out]
        n331 = Array Subset(array=w428, length=99) -> (w430:string[])  [unwired: 1 in]
        n332 = Build Array (concatenate)(w433, w430) -> (w431:string[])
        n333 = local write "User Message"(w423) -> ()
        n334 = call "PDP Log Message.vi"("Message"=w423) -> ()
        n335 = property on="Previous Messages" class="Ring (strict)"("Strings []"=w431) -> ()  [unwired: 2 in, 2 out]
        n336 = property on="Error" class="Bool (strict)"("Blinking"=TRUE) -> ()  [unwired: 2 in, 2 out]
        n337 = property on="User Message" class="Str"("Text.Text Colors:Text Color"=u32 16711680) -> ()  [unwired: 2 in, 2 out]
      }
      frame "Address=" {
        n338 = Scan From String(format string="%3s,%[.0-9]:%d" ("Format String"), input string=w438) -> (output 1=w436:string, output 2=w437:string, output 3=w435:i32)  [unwired: 5 in, 3 out]
        n339 = call "Message Set Module Address.vi"("Port"=w435, "Address"=w437, "Module"=w436) -> ()
      }
      frame "Stop" {
        n340 = Stop() -> ()  [unwired: 1 in]
      }
    }
  }
  n341 = stacked-sequence "Process Button Presses" {
    frame #0 {
      w440 = TRUE ("X Editable")
      # "Check that the path global has been set."
      # "Perform any necessary startup functions."
      n342 = global read "TPS Global.vi" "TPS Base Path"() -> (w444:path)
      n343 = local write "User Message"("") -> ()
      n344 = property on="Subtracted Signal & PolyFit Curve" class="XYGraph (strict)"("X Scale.Editable"=w440) -> ()  [unwired: 2 in, 2 out]
      n345 = property on="Polysub Signal" class="XYGraph (strict)"("X Scale.Editable"=w440) -> ()  [unwired: 2 in, 2 out]
      n346 = Not A Number/Path/Refnum?(number/path/refnum=w444) -> (NaN/Path/Refnum?=w445:bool)
      n347 = case shown="False" w445 {
        tunnel: w444 -> [w460 _]
        frame False {
          n348 = global read "TPS Global.vi" "TPS Setup File"() -> (w468:string)
          n349 = Build Path(base path=w460, name or relative path=w468) -> (appended path=w467:path)
          n350 = call <vilib>:"Open Config Data (compatibility).vi"("create file if necessary (T)"=FALSE ("create file if necessary? (T)"), "configuration file path"=w467) -> ("error out"=w469:errorcluster, "refnum"=w465:T4)  [unwired: 7 in, 1 out]
          n351 = call-poly <vilib>:"Read Key.vi"("section"="PDP", "error in (no error)"=w469, "default value"=path "", "key"="Message Log", "refnum"=w465) -> ("error out"=w470:errorcluster, "value"=w459:path, "refnum out"=w461:T4)  [unwired: 3 in, 1 out]
          n352 = call <vilib>:"Close Config Data.vi"("error in (no error)"=w470, "write file if changed (T)"=FALSE, "refnum"=w461) -> ("error out"=w471:errorcluster)  [unwired: 7 in, 1 out]
          n353 = Build Path(base path=w460, name or relative path=w459) -> (appended path=w458:path)
          n354 = global write "PDP Global.vi" "Message Log"(w458) -> ()
          n355 = call <vilib>:"Simple Error Handler.vi"("error in (no error)"=w471) -> ()  [unwired: 4 in, 5 out]
        }
        frame True {
          n356 = One Button Dialog(message="The Base Path global has not been set.  Please set it and run again.") -> (true=w473:bool)  [unwired: 1 in]
          n357 = Stop(stop? (T)=w473) -> ()
        }
      }
      n358 = call "Message Send.vi"("Message"="Read", "Destination"="SMC") -> ()
      n359 = case shown="True" "Case Constant\n(See Context Help)" {
        frame False {
        }
        frame True {
          n360 = global read "TMC Global.vi" "Status Chans"() -> (w455:string)
          n361 = global read "TMC Global.vi" "Target Mover Device"() -> (w456:i32)
          n362 = Spreadsheet String To Array(delimiter (Tab)=",", format string="%d", spreadsheet string=w455, array type (2D Dbl)=i32[] [] ("Array Constant")) -> (array=w452:i32[])
          n363 = call "DIO Read.vi"("Channels"=w452, "device"=w456) -> ("Data"=w450:bool[])  [unwired: 1 out]
          n364 = Boolean Array To Number(Boolean array=w450) -> (number=w449:u32)
          n365 = call "Encoder Read.vi"() -> ("Encoder Position"=w447:dbl)
          n366 = Decrement(x=w449) -> (x-1=w448:u32)
          n367 = local write "Encoder"(w447) -> ()
          n368 = local write "Target Pos"(w448) -> ()
        }
      }
    }
    frame #1 {
      n369 = while {
        stop <- FALSE stop-if-true
        n370 = event shown="[18] \"Sweeps\": Value Change" {
          selector: _ -> [_ _ _ _ _ _ _ _ _ _ _ _ _ _ _ _ _ _ _ _ _ _ _ _ _ _ _ _ _ _ _ _ _ _ _ _ _ _ _ _ _ _ _ _ _ _ _ _]
          dyn-events: _ -> [_ _ _ _ _ _ _ _ _ _ _ _ _ _ _ _ _ _ _ _ _ _ _ _ _ _ _ _ _ _ _ _ _ _ _ _ _ _ _ _ _ _ _ _ _ _ _ _]
          timeout: 1000 -> [_ _ _ _ _ _ _ _ _ _ _ _ _ _ _ _ _ _ _ _ _ _ _ _ _ _ _ _ _ _ _ _ _ _ _ _ _ _ _ _ _ _ _ _ _ _ _ _]
          event "Init QCA": Value Change {
            n371 = event-data() -> ()  [unwired: 1 in, 4 out]
            n372 = call "Message Send.vi"("Message"="Init", "Destination"="QCA") -> ()
          }
          event "Save Channel List": Value Change {
            n373 = event-data() -> ()  [unwired: 1 in, 4 out]
            n374 = call "Message Send.vi"("Message"="SaveChans", "Destination"="QCA") -> ()
          }
          event "Stop NMR Sweep": Value Change {
            n375 = event-data() -> ()  [unwired: 1 in, 5 out]
            n376 = call "Stop NMR Sweep.vi"() -> ()  [unwired: 1 in]
          }
          event "DC Convert": Value Change {
            n377 = event-data() -> ()  [unwired: 1 in, 5 out]
            n378 = call "Yale DC Convert.vi"() -> ()  [unwired: 1 in]
          }
          event "Baseline": Value Change {
            n379 = event-data() -> ()  [unwired: 1 in, 4 out]
            n380 = call "Message Send.vi"("Message"="Baseline", "Destination"="QCA") -> ()
          }
          event "Pause": Value Change {
            n381 = event-data() -> ()  [unwired: 1 in, 4 out]
            n382 = call "Message Send.vi"("Message"="Pause", "Destination"="QCA") -> ()
          }
          event "Take Data": Value Change {
            n383 = event-data() -> ()  [unwired: 1 in, 4 out]
            n384 = call "Message Send.vi"("Message"="TakeData", "Destination"="QCA") -> ()
          }
          event "One Point": Value Change {
            n385 = event-data() -> ()  [unwired: 1 in, 4 out]
            n386 = call "Message Send.vi"("Message"="OnePoint", "Destination"="QCA") -> ()
          }
          event "NMR Tune": Value Change {
            n387 = event-data() -> ()  [unwired: 1 in, 4 out]
            n388 = call "Message Send.vi"("Message"="NMRTune", "Destination"="QCA") -> ()
          }
          event "Monitor": Value Change {
            n389 = event-data() -> ()  [unwired: 1 in, 4 out]
            n390 = call "Message Send.vi"("Message"="Monitor", "Destination"="QCA") -> ()
          }
          event "ScanSteps": Value Change {
            n391 = event-data() -> ("NewVal"=w492:i32)  [unwired: 1 in, 4 out]
            n392 = call "Message Send Integer.vi"("Value"=w492, "Parameter"="ScanSteps" ("Message"), "Destination"="QCA") -> ()
          }
          event "Scan Freq": Value Change {
            n393 = event-data() -> ("NewVal"=w495:i32)  [unwired: 1 in, 4 out]
            n394 = call "Message Send Integer.vi"("Value"=w495, "Parameter"="ScanFreq" ("Message"), "Destination"="QCA") -> ()
          }
          event "RF On": Value Change {
            n395 = event-data() -> ()  [unwired: 1 in, 5 out]
            n396 = call "Message Send.vi"("Message"="RF On", "Destination"="QCA") -> ()
          }
          event "RF Off": Value Change {
            n397 = event-data() -> ()  [unwired: 1 in, 5 out]
            n398 = call "Message Send.vi"("Message"="RF Off", "Destination"="QCA") -> ()
          }
          event "RF Freq": Value Change {
            n399 = event-data() -> ("NewVal"=w502:dbl)  [unwired: 1 in, 4 out]
            n400 = call "Message Send Float.vi"("Value"=w502, "Parameter"="RFFreq" ("Message"), "Destination"="QCA") -> ()
          }
          event "RF Mod": Value Change {
            n401 = event-data() -> ("NewVal"=w505:i32)  [unwired: 1 in, 4 out]
            n402 = call "Message Send Integer.vi"("Value"=w505, "Parameter"="RFMod" ("Message"), "Destination"="QCA") -> ()
          }
          event "RF Power": Value Change {
            n403 = event-data() -> ("NewVal"=w508:i32)  [unwired: 1 in, 4 out]
            n404 = call "Message Send Integer.vi"("Value"=w508, "Parameter"="RFPower" ("Message"), "Destination"="QCA") -> ()
          }
          event "NMR Channel": Value Change {
            n405 = event-data() -> ("NewVal"=w511:i32)  [unwired: 1 in, 4 out]
            n406 = call "Message Send Integer.vi"("Value"=w511, "Parameter"="Channel" ("Message"), "Destination"="QCA") -> ()
          }
          event "Sweeps": Value Change {
            n407 = event-data() -> ("NewVal"=w514:i32)  [unwired: 1 in, 4 out]
            n408 = call "Message Send Integer.vi"("Value"=w514, "Parameter"="ScanSweeps" ("Message"), "Destination"="QCA") -> ()
          }
          event "Cal. Const.": Value Change {
            n409 = event-data() -> ("NewVal"=w517:dbl)  [unwired: 1 in, 4 out]
            n410 = call "Message Send Float.vi"("Value"=w517, "Parameter"="CalConst" ("Message"), "Destination"="QCA") -> ()
          }
          event "Yale Gain": Value Change {
            n411 = event-data() -> ("NewVal"=w520:i32)  [unwired: 1 in, 4 out]
            n412 = call "Message Send Integer.vi"("Value"=w520, "Parameter"="YaleGain" ("Message"), "Destination"="QCA") -> ()
          }
          event "Mon. Time": Value Change {
            n413 = event-data() -> ("NewVal"=w523:i32)  [unwired: 1 in, 4 out]
            n414 = call "Message Send Integer.vi"("Value"=w523, "Parameter"="MonitorDelay" ("Message"), "Destination"="QCA") -> ()
          }
          event "SetPoint (A)": Value Change {
            n415 = event-data() -> ("NewVal"=w526:dbl)  [unwired: 1 in, 4 out]
            n416 = call "Message Send Float.vi"("Value"=w526, "Parameter"="Setpoint" ("Message"), "Destination"="SMC") -> ()
          }
          event "Rate (A/min)": Value Change {
            n417 = event-data() -> ("NewVal"=w529:dbl)  [unwired: 1 in, 4 out]
            n418 = call "Message Send Float.vi"("Value"=w529, "Parameter"="Setrate" ("Message"), "Destination"="SMC") -> ()
          }
          event "FM Amplitude (V)": Value Change {
            n419 = event-data() -> ("NewVal"=w532:dbl)  [unwired: 1 in, 4 out]
            n420 = call "Message Send Float.vi"("Value"=w532, "Parameter"="FMAmplitude" ("Message"), "Destination"="MWC") -> ()
          }
          event "FM Offset (V)": Value Change {
            n421 = event-data() -> ("NewVal"=w535:dbl)  [unwired: 1 in, 4 out]
            n422 = call "Message Send Float.vi"("Value"=w535, "Parameter"="FMOffset" ("Message"), "Destination"="MWC") -> ()
          }
          event "Switch Heater On": Value Change {
            n423 = event-data() -> ()  [unwired: 1 in, 5 out]
            n424 = call "Message Send Text.vi"("Value"="On", "Parameter"="Heater" ("Message"), "Destination"="SMC") -> ()
          }
          event "Switch Heater Off": Value Change {
            n425 = event-data() -> ()  [unwired: 1 in, 5 out]
            n426 = call "Message Send Text.vi"("Value"="Off", "Parameter"="Heater" ("Message"), "Destination"="SMC") -> ()
          }
          event "Hold": Value Change {
            n427 = event-data() -> ()  [unwired: 1 in, 5 out]
            n428 = call "Message Send Text.vi"("Value"="Hold", "Parameter"="MagStatus" ("Message"), "Destination"="SMC") -> ()
          }
          event "To Setpoint": Value Change {
            n429 = event-data() -> ()  [unwired: 1 in, 5 out]
            n430 = call "Message Send Text.vi"("Value"="To Setpoint", "Parameter"="MagStatus" ("Message"), "Destination"="SMC") -> ()
          }
          event "To Zero": Value Change {
            n431 = event-data() -> ()  [unwired: 1 in, 5 out]
            n432 = call "Message Send Text.vi"("Value"="To Zero", "Parameter"="MagStatus" ("Message"), "Destination"="SMC") -> ()
          }
          event "Magnet Lockout": Value Change {
            n433 = event-data() -> ()  [unwired: 1 in, 5 out]
            n434 = call "Message Send.vi"("Message"="Control" ("Value"), "Destination"="SMC") -> ()
          }
          event "He4 Range": Value Change {
            n435 = event-data() -> ("NewVal"=w555:i32)  [unwired: 1 in, 4 out]
            n436 = call "Message Send Integer.vi"("Value"=w555, "Parameter"="He4Range", "Destination"="TTM") -> ()
          }
          event "Enable TCL Buttons": Value Change {
            w559 = string[] ["Disable Buttons", "Disable Buttons", "Disable Buttons", "Disable Buttons"] ("Array Constant")
            n437 = event-data() -> ()  [unwired: 1 in, 5 out]
            n438 = property on="Enable TCL Buttons" class="Bool"() -> ("Strings [4]"=w562:string[])  [unwired: 2 in, 2 out]
            n439 = Equal?(x=w562, y=w559) -> (x = y?=w561:bool)
            n440 = Select(t=string[] ["Enable Buttons", "Enable Buttons", "Enable Buttons", "Enable Buttons"] ("Array Constant"), s=w561, f=w559) -> (s? t:f=w565:string[])
            n441 = Select(t=2, s=w561, f=0) -> (s? t:f=w558:i32)
            n442 = property on="Enable TCL Buttons" class="Bool"("Strings [4]"=w565) -> ()  [unwired: 2 in, 2 out]
            n443 = property on="NewEventFile" class="Bool"("Disabled"=w558) -> ()  [unwired: 2 in, 2 out]
            n444 = property on="NewBaseFile" class="Bool"("Disabled"=w558) -> ()  [unwired: 2 in, 2 out]
          }
          event "NewEventFile": Value Change {
            n445 = event-data() -> ()  [unwired: 1 in, 5 out]
            n446 = property on="NewBaseFile" class="Bool"() -> ("Disabled"=w567:u8)  [unwired: 2 in, 2 out]
            n447 = Equal To 0?(x=w567) -> (x = 0?=w566:bool)
            n448 = case shown="True" w566 {
              frame False {
              }
              frame True {
                n449 = call "Message Send.vi"("Message"="NewEventFile", "Destination"="TCL") -> ()
              }
            }
          }
          event "NewBaseFile": Value Change {
            n450 = event-data() -> ()  [unwired: 1 in, 5 out]
            n451 = property on="NewBaseFile" class="Bool"() -> ("Disabled"=w571:u8)  [unwired: 2 in, 2 out]
            n452 = Equal To 0?(x=w571) -> (x = 0?=w570:bool)
            n453 = case shown="True" w570 {
              frame False {
              }
              frame True {
                n454 = call "Message Send.vi"("Message"="NewBaseFile", "Destination"="TCL") -> ()
              }
            }
          }
          event "Error": Value Change {
            w575 = FALSE ("Blinking")
            n455 = event-data() -> ()  [unwired: 1 in, 5 out]
            n456 = local write "Error"(w575) -> ()
            n457 = property on="Error" class="Bool (strict)"("Blinking"=w575) -> ()  [unwired: 2 in, 2 out]
            "User Message" <- ""
          }
          event "5 min": Value Change {
            n458 = event-data() -> ()  [unwired: 1 in, 5 out]
            n459 = property on="History Plot" class="XYGraph (strict)"() -> ("X Scale.Range:Maximum"=w578:dbl)  [unwired: 2 in, 2 out]
            n460 = Subtract(x=w578, y=300) -> (x-y=w577:dbl)
            n461 = property on="History Plot" class="XYGraph (strict)"("X Scale.Range:Minimum"=w577) -> ()  [unwired: 2 in, 2 out]
          }
          event "15 min": Value Change {
            n462 = event-data() -> ()  [unwired: 1 in, 5 out]
            n463 = property on="History Plot" class="XYGraph (strict)"() -> ("X Scale.Range:Maximum"=w581:dbl)  [unwired: 2 in, 2 out]
            n464 = Subtract(x=w581, y=900) -> (x-y=w580:dbl)
            n465 = property on="History Plot" class="XYGraph (strict)"("X Scale.Range:Minimum"=w580) -> ()  [unwired: 2 in, 2 out]
          }
          event "30 min": Value Change {
            n466 = event-data() -> ()  [unwired: 1 in, 5 out]
            n467 = property on="History Plot" class="XYGraph (strict)"() -> ("X Scale.Range:Maximum"=w584:dbl)  [unwired: 2 in, 2 out]
            n468 = Subtract(x=w584, y=1800) -> (x-y=w583:dbl)
            n469 = property on="History Plot" class="XYGraph (strict)"("X Scale.Range:Minimum"=w583) -> ()  [unwired: 2 in, 2 out]
          }
          event "+1 hour": Value Change {
            n470 = event-data() -> ()  [unwired: 1 in, 5 out]
            n471 = property on="History Plot" class="XYGraph (strict)"() -> ("X Scale.Range:Minimum"=w587:dbl)  [unwired: 2 in, 2 out]
            n472 = Subtract(x=w587, y=3600) -> (x-y=w586:dbl)
            n473 = property on="History Plot" class="XYGraph (strict)"("X Scale.Range:Minimum"=w586) -> ()  [unwired: 2 in, 2 out]
          }
          event "Increase": Value Change {
            n474 = event-data() -> ()  [unwired: 1 in, 5 out]
            n475 = property on="History Plot" class="XYGraph (strict)"() -> ("Y Scale.Range:Maximum"=w591:dbl, "Y Scale.Range:Minimum"=w592:dbl)  [unwired: 2 in, 2 out]
            n476 = Subtract(x=w591, y=w592) -> (x-y=w589:dbl)
            n477 = Divide(x=w589, y=2) -> (x/y=w588:dbl)
            n478 = Add(x=w591, y=w588) -> (x+y=w593:dbl)
            n479 = Subtract(x=w592, y=w588) -> (x-y=w594:dbl)
            n480 = property on="History Plot" class="XYGraph (strict)"("Y Scale.Range:Maximum"=w593, "Y Scale.Range:Minimum"=w594) -> ()  [unwired: 2 in, 2 out]
          }
          event "Decrease": Value Change {
            n481 = event-data() -> ()  [unwired: 1 in, 5 out]
            n482 = property on="History Plot" class="XYGraph (strict)"() -> ("Y Scale.Range:Maximum"=w598:dbl, "Y Scale.Range:Minimum"=w599:dbl)  [unwired: 2 in, 2 out]
            n483 = Subtract(x=w598, y=w599) -> (x-y=w596:dbl)
            n484 = Divide(x=w596, y=4) -> (x/y=w595:dbl)
            n485 = Subtract(x=w598, y=w595) -> (x-y=w600:dbl)
            n486 = Add(x=w599, y=w595) -> (x+y=w601:dbl)
            n487 = property on="History Plot" class="XYGraph (strict)"("Y Scale.Range:Maximum"=w600, "Y Scale.Range:Minimum"=w601) -> ()  [unwired: 2 in, 2 out]
          }
          event "Up": Value Change {
            n488 = event-data() -> ()  [unwired: 1 in, 5 out]
            n489 = property on="History Plot" class="XYGraph (strict)"() -> ("Y Scale.Range:Maximum"=w605:dbl, "Y Scale.Range:Minimum"=w606:dbl)  [unwired: 2 in, 2 out]
            n490 = Subtract(x=w605, y=w606) -> (x-y=w603:dbl)
            n491 = Divide(x=w603, y=4) -> (x/y=w602:dbl)
            n492 = Add(x=w605, y=w602) -> (x+y=w607:dbl)
            n493 = Add(x=w606, y=w602) -> (x+y=w608:dbl)
            n494 = property on="History Plot" class="XYGraph (strict)"("Y Scale.Range:Maximum"=w607, "Y Scale.Range:Minimum"=w608) -> ()  [unwired: 2 in, 2 out]
          }
          event "Down": Value Change {
            n495 = event-data() -> ()  [unwired: 1 in, 5 out]
            n496 = property on="History Plot" class="XYGraph (strict)"() -> ("Y Scale.Range:Maximum"=w612:dbl, "Y Scale.Range:Minimum"=w613:dbl)  [unwired: 2 in, 2 out]
            n497 = Subtract(x=w612, y=w613) -> (x-y=w610:dbl)
            n498 = Divide(x=w610, y=4) -> (x/y=w609:dbl)
            n499 = Subtract(x=w612, y=w609) -> (x-y=w614:dbl)
            n500 = Subtract(x=w613, y=w609) -> (x-y=w615:dbl)
            n501 = property on="History Plot" class="XYGraph (strict)"("Y Scale.Range:Maximum"=w614, "Y Scale.Range:Minimum"=w615) -> ()  [unwired: 2 in, 2 out]
          }
          event "Submit Comment": Value Change {
            n502 = event-data() -> ()  [unwired: 1 in, 5 out]
            n503 = stacked-sequence {
              frame #0 {
                n504 = call "PDP Send User Comment.vi"("User Comment (press submit when done)") -> ()
              }
              frame #1 {
                n505 = local write "User Comment (press submit when done)"("") -> ()
              }
            }
          }
          event "Move Target": Value Change {
            n506 = event-data() -> ()  [unwired: 1 in, 5 out]
            n507 = call "TMC.vi"() -> ("Position"=w618:u32, "Encoder Readout"=→"Encoder":dbl)
            n508 = Decrement(x=w618) -> (x-1=→"Target Pos":u32)
          }
          event Timeout {
            n509 = local read "Clear Message Time"() -> (w623:i32)
            n510 = event-data() -> ()  [unwired: 1 in, 2 out]
            n511 = call "Get UNIX Time.vi"() -> ("UNIX seconds"=w621:i32)
            n512 = local read "Update At (sec)"() -> (w628:i32)
            n513 = Greater Or Equal?(x=w621, y=w623) -> (x >= y?=w622:bool)
            n514 = Subtract(x=w628, y=w621) -> (x-y=w627:i32)
            n515 = case shown="True" w622 {
              frame False {
              }
              frame True {
                n516 = local write "User Message"("") -> ()
              }
            }
            n517 = Greater Or Equal To 0?(x=w627) -> (x >= 0?=w626:bool)
            n518 = case shown="False" w626 {
              tunnel: w627 -> [_ w639]
              frame False {
                n519 = local read "NMR Tune Light"() -> (w637:bool)
                n520 = local read "Pause Light"() -> (w636:bool)
                n521 = Not Or(1:w637, 2:w636) -> (0:w638:bool)
                n522 = property on="Next Update" class="DigNum (strict)"("Visible"=w638) -> ()  [unwired: 2 in, 2 out]
              }
              frame True {
                "Next Update" <- w639
              }
            }
            n523 = property on="Heater Delay" class="DigNum (strict)"() -> ("Visible"=w624:bool)  [unwired: 2 in, 2 out]
            n524 = case shown="True" w624 {
              frame False {
              }
              frame True {
                n525 = Get Date/Time In Seconds() -> (seconds since 1Jan1904=w630:timestamp)
                n526 = To Double Precision Float(number=w630) -> (double precision float=w632:dbl)
                n527 = Subtract(x="Heater Delay Done", y=w632) -> (x-y=w631:dbl)
                "Heater Delay" <- w631
                n528 = Less Or Equal To 0?(x=w631) -> (x <= 0?=w635:bool)
                n529 = Not(x=w635) -> (.not. x?=w634:bool)
                n530 = property on="Switch Heater On" class="Bool"("Visible"=w635) -> ()  [unwired: 2 in, 2 out]
                n531 = property on="Switch Heater Off" class="Bool"("Visible"=w635) -> ()  [unwired: 2 in, 2 out]
                n532 = property on="Heater Delay" class="DigNum (strict)"("Visible"=w634) -> ()  [unwired: 2 in, 2 out]
              }
            }
            n533 = property on="Error" class="Bool (strict)"() -> ("Blinking"=w625:bool)  [unwired: 2 in, 2 out]
            n534 = case shown="True" w625 {
              frame False {
              }
              frame True {
                n535 = call <vilib>:"Beep.vi"() -> ()  [unwired: 12 in]
              }
            }
          }
        }
      }
    }
    frame #2 {
    }
  }
